vi "ChoosePickupAddress.vi"(8 "error in (no error)":errorcluster, 10 "Sender Data":T1, 11 "Post in":refnum<class "Post.lvclass">) -> (0 "error out":errorcluster, 3 "Post out":refnum<class "Post.lvclass">)   [LabVIEW 2019, in "Post.lvclass"]
uses:
  Post.lvclass
  C:/Users/Extensa/Desktop/Fabryka/Fabryka Rozwiazanie/Delivery/Delivery/Delivery.lvclass
  Controls/#cluster_PersonalData.ctl
  Post.lvclass/Post.ctl
  Delivery/Delivery.lvclass/Delivery.ctl
  Delivery/Delivery.lvclass
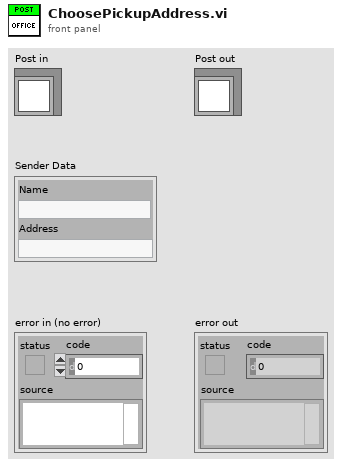
[diagram p1: front panel]
types:
  T1 = typedef "#cluster_PersonalData.ctl" = cluster{"Name":string, "Address":string}
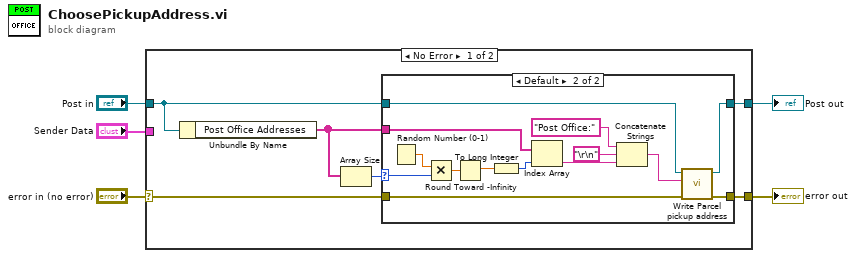
[diagram p0: block diagram]
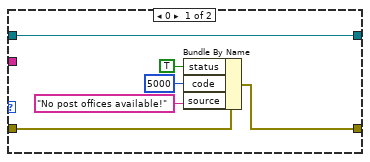
[diagram p2: hidden frame]
diagram:
  n1 = case shown="No Error" "error in (no error)" {
    selector: "error in (no error)" -> [w11 w33]
    tunnel: [w10 w33] -> w4
    tunnel: [w9 w32] -> w2
    tunnel: "Post in" -> [w8 w32]
    tunnel: "Sender Data" -> [_ _]
    frame No Error {
      n2 = Unbundle By Name(w8) -> ("Post Office Addresses"=w6:string[])
      n3 = Array Size(array=w6) -> (size(s)=w7:i32)
      n4 = case shown="Default" w7 {
        selector: w7 -> [_ w21]
        tunnel: w11 -> [w16 w31]
        tunnel: [w15 w30] -> w10
        tunnel: [w17 w29] -> w9
        tunnel: w8 -> [w17 w24]
        tunnel: w6 -> [_ w23]
        frame 0 {
          n5 = Bundle By Name(cluster=w16, "status"=TRUE, "code"=5000, "source"="No post offices available!") -> (w15:errorcluster)
        }
        frame Default {
          n6 = Random Number (0-1)() -> (number: 0 to 1=w22:dbl)
          n7 = Multiply(x=w22, y=w21) -> (x*y=w20:dbl)
          n8 = Round Toward -Infinity(1:w20) -> (0:w18:dbl)
          n9 = To Long Integer(number=w18) -> (32bit integer=w19:i32)
          n10 = Index Array(array=w23, index=w19) -> (element=w27:string)
          n11 = Concatenate Strings("Post Office:" ("string"), "\r\n", w27) -> (w25:string)
          n12 = call "Write Parcel pickup address.vi"("error in (no error)"=w31, "Parcel pickup address"=w25, "Delivery in"=w24) -> ("error out"=w30:errorcluster, "Delivery out"=w29:refnum<class "Post.lvclass">)  [unwired: 7 in]
        }
      }
    }
    frame Error {
    }
  }
  "error out" <- w4
  "Post out" <- w2
